vi "controlAQuadBInResolution.vi"(6 "Set":bool, 7 "error in":errorcluster, 8 "Resolution in":i32, 9 "axis in":u8, 10 "connection ID":i32) -> (0 "error out":errorcluster, 1 "Resolution out":i32, 2 "axis out":u8, 3 "connection ID":i32)   [LabVIEW 2016]
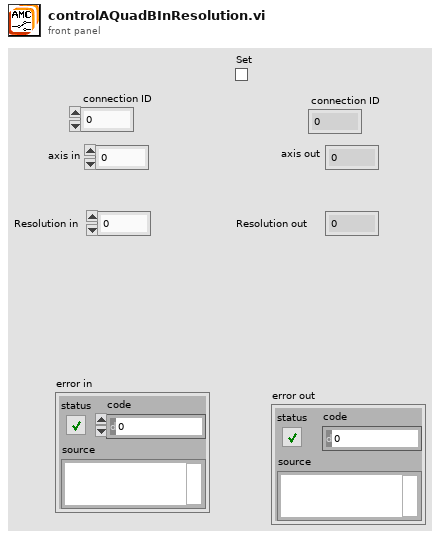
[diagram p1: front panel]
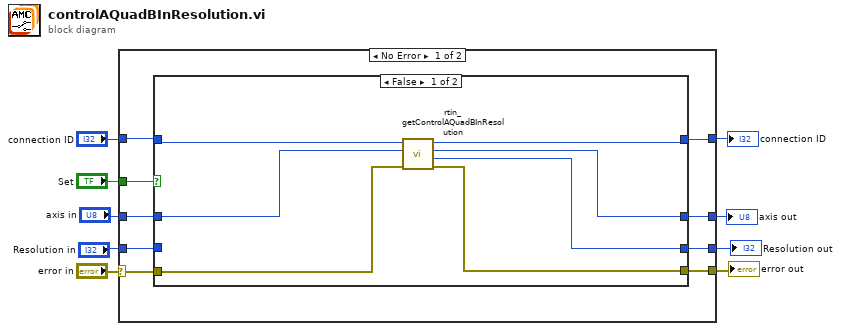
[diagram p0: block diagram]
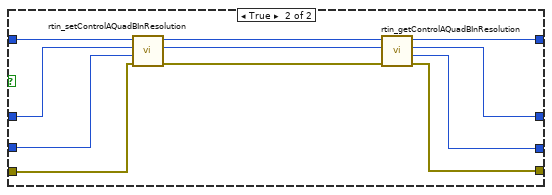
[diagram p2: hidden frame]
diagram:
  n1 = case shown="No Error" "error in" {
    selector: "error in" -> [w12 w40]
    tunnel: "axis in" -> [w16 w38]
    tunnel: [w14 w40] -> w8
    tunnel: [w11 w38] -> w7
    tunnel: "Set" -> [w13 _]
    tunnel: [w17 w37] -> w5
    tunnel: "connection ID" -> [w18 w37]
    tunnel: "Resolution in" -> [w15 w39]
    tunnel: [w10 w39] -> w3
    frame No Error {
      n2 = case shown="False" w13 {
        tunnel: [w24 w31] -> w17
        tunnel: w18 -> [w25 w36]
        tunnel: w16 -> [w21 w35]
        tunnel: [w22 w28] -> w14
        tunnel: w15 -> [_ w34]
        tunnel: w12 -> [w23 w33]
        tunnel: [w20 w26] -> w11
        tunnel: [w19 w27] -> w10
        frame False {
          n3 = call "rtin_getControlAQuadBInResolution.vi"("error in"=w23, "axis"=w21, "connection ID"=w25) -> ("error out"=w22:errorcluster, "resolution"=w19:i32, "axis_out"=w20:i32, "connection ID"=w24:i32)  [unwired: 5 in]
        }
        frame True {
          n4 = call "rtin_setControlAQuadBInResolution.vi"("error in"=w33, "resolution"=w34, "axis"=w35, "connection ID"=w36) -> ("error out"=w29:errorcluster, "axis_out"=w30:i32, "connection ID"=w32:i32)  [unwired: 5 in]
          n5 = call "rtin_getControlAQuadBInResolution.vi"("error in"=w29, "axis"=w30, "connection ID"=w32) -> ("error out"=w28:errorcluster, "resolution"=w27:i32, "axis_out"=w26:i32, "connection ID"=w31:i32)  [unwired: 5 in]
        }
      }
    }
    frame Error {
    }
  }
  "error out" <- w8
  "axis out" <- w7
  "connection ID" <- w5
  "Resolution out" <- w3
